vi "VICI Electronic Actuator Test.vi"() -> ()   [LabVIEW 2018, in "VICI Electronic Actuator.lvlib"]
uses:
  D-O Module Folder/DIO Valve/VICI Electronic Actuator.lvlib
  VICI Electronic Actuator Settings.ctl
  <vilib>/Platform/TimedLoop/XDataNode/timing_clust.ctl
  <vilib>/Platform/TimedLoop/XDataNode/nitl_modes.ctl
  <vilib>/Platform/TimedLoop/XDataNode/wakeup.ctl
  <vilib>/Platform/TimedLoop/XDataNode/XDataNode.xnode
  <vilib>/Platform/TimedLoop/XDataNode/XDNodeRunTimeDep.lvlib
panel:
  in  "stop":bool
  in  "VICI Electronic Actuator":T1
  in  "Period":i64
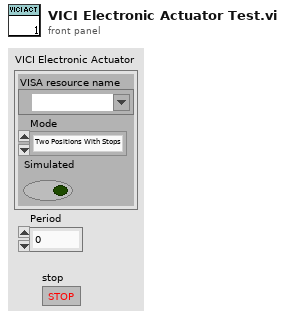
[diagram p1: front panel]
types:
  T1 = typedef "VICI Electronic Actuator.lvlib/VICI Electronic Actuator Settings.ctl" = cluster{"VISA resource name":refnum<visa-resource-name>, "Mode":enum16{"Two Positions With Stops", "Two Positions Without Stops", "Mutiposition"}, "Simulated":bool}
  T2 = typedef "XDNodeRunTimeDep.lvlib/timing_clust.ctl" = cluster{"Expected End [f-1]":u64, "Actual End [f-1]":u64, "Finished Late? [f-1]":bool, "Expected End [i-1]":u64, "Actual End [i-1]":u64, "Finished Late? [i-1]":bool, "Expected Start [i]":u64, "Actual Start [i]":u64, "Expected Start [f]":u64, "Actual Start [f]":u64, "Source Name":string, "Structure Name":string, "Period":i64, "Deadline":i64, "Offset":i64, "Start":i64, "Priority":i32, "Timeout":i32, "Mode":T3, "Wakeup Reason":T4, "Error":errorcluster, "Source Type":string, "Secondary Source Type":string, "Global End Time":u64, "Global Start Time":u64, "Frame Duration":u64, "Iteration Duration":u64, "Assigned CPU":i32, "I/O Scan Engine Mode":u32}
  T3 = typedef "XDNodeRunTimeDep.lvlib/nitl_modes.ctl" = enum32{"No Change", "Process missed periods, maintain original phase", "Discard missed periods, maintain original phase", "Process missed periods, ignore original phase", "Discard missed periods, ignore original phase"}
  T4 = typedef "XDNodeRunTimeDep.lvlib/wakeup.ctl" = enum32{"Normal", "Aborted", "Asynchronous wakeup", "Timing source error", "Timed loop error", "Timeout"}
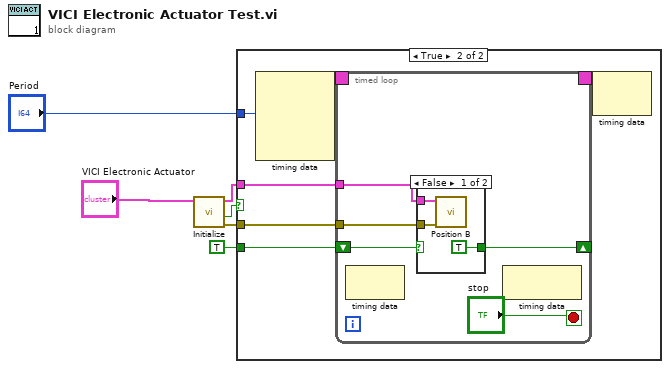
[diagram p0: block diagram]
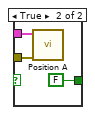
[diagram p3: hidden frame]
diagram:
  n1 = call "Initialize.vi"("VICI Electronic Actuator In"="VICI Electronic Actuator") -> ("error out"=w3:errorcluster, "Initialized"=w2:bool, "VICI Electronic Actuator Out"=w4:T1)  [unwired: 7 in, 1 out]
  n2 = case shown="True" w2 {
    tunnel: "Period" -> [_ w10]
    tunnel: TRUE -> [_ w9]
    tunnel: w4 -> [_ w8]
    tunnel: w3 -> [_ w7]
    frame False {
    }
    frame True {
      n3 = node-c288(w10) -> (w12:T2)  [unwired: 3 in]
      n4 = timed-loop {
        timing: w12 -> [_]
        timing-out: [_] -> w11
        shift-right: [w17] -> _
        shift-left: w9 -> [w16]
        tunnel: w8 -> [w15]
        tunnel: w7 -> [w14]
        stop <- "stop" stop-if-true
        n5 = node-c288() -> ()  [unwired: 1 in, 1 out]
        n6 = case shown="False" w16 {
          tunnel: [TRUE FALSE] -> w17
          tunnel: w15 -> [w19 w22]
          tunnel: w14 -> [w20 w21]
          frame False {
            n7 = call "Position B.vi"("error in (no error)"=w20, "VICI Electronic Actuator In"=w19) -> ()  [unwired: 7 in, 3 out]
          }
          frame True {
            n8 = call "Position A.vi"("error in (no error)"=w21, "VICI Electronic Actuator In"=w22) -> ()  [unwired: 6 in, 4 out]
          }
        }
        n9 = node-c288() -> ()  [unwired: 1 in, 1 out]
      }
      n10 = node-c288(w11) -> ()  [unwired: 1 out]
    }
  }
